vi "SoundIF.vi"(8 "Numeric":dbl) -> (0 "Boolean":bool)   [LabVIEW 2019]
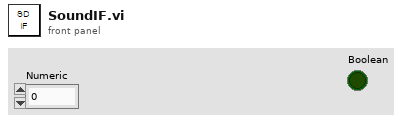
[diagram p1: front panel]
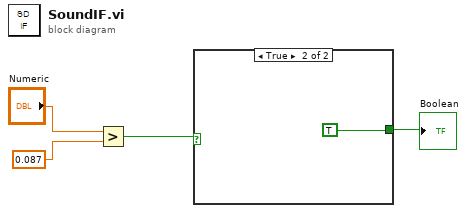
[diagram p0: block diagram]
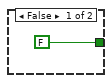
[diagram p2: hidden frame]
diagram:
  n1 = Greater?(x="Numeric", y=0.087 ("x")) -> (0:w4:bool)
  n2 = case shown="True" w4 {
    tunnel: [FALSE TRUE] -> w3
    frame False {
    }
    frame True {
    }
  }
  "Boolean" <- w3
